vi "Write NewTestRole.vi"(8 "error in (no error)":errorcluster, 10 "NewTestRole.lvclass":refnum<class "NewTestRole.lvclass">, 11 "KeeperPlay in":refnum<class "KeeperPlay.lvclass">) -> (0 "error out":errorcluster, 3 "KeeperPlay out":refnum<class "KeeperPlay.lvclass">)   [LabVIEW 2022 SP3, in "KeeperPlay.lvclass"]
uses:
  KeeperPlay.lvclass
  NewTestRole/NewTestRole.lvclass
  KeeperPlay.lvclass/KeeperPlay.ctl
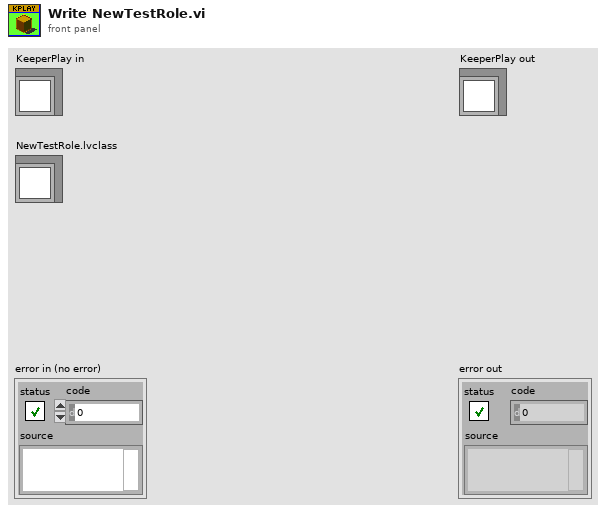
[diagram p1: front panel]
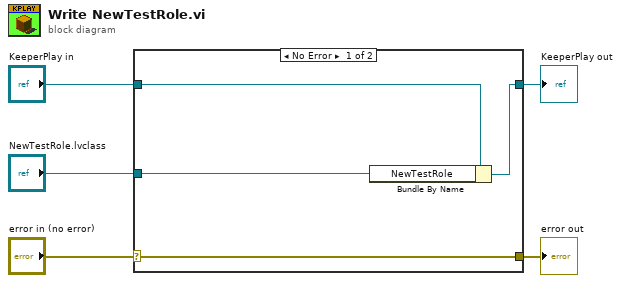
[diagram p0: block diagram]
diagram:
  n1 = case shown="No Error" "error in (no error)" {
    selector: "error in (no error)" -> [w9 w10]
    tunnel: [w9 w10] -> w4
    tunnel: [w7 w11] -> w2
    tunnel: "KeeperPlay in" -> [w8 w11]
    tunnel: "NewTestRole.lvclass" -> [w6 _]
    frame No Error {
      n2 = Bundle By Name(cluster=w8, "NewTestRole"=w6) -> (w7:refnum<class "KeeperPlay.lvclass">)
    }
    frame Error {
    }
  }
  "error out" <- w4
  "KeeperPlay out" <- w2
